vi "数据存储接口.vi"(4 "快捷测试？":bool, 5 "质控参数设置":T1, 6 "标样校准？":bool, 7 "数据标记表":string, 8 "空白校准？":bool, 10 "数据存储模式":T2(ring), 11 "测量数据区":T4) -> (2 "x != y?":bool, 3 "data输出":T3)   [LabVIEW 2016, in "斯坦道总磷总氮.lvlib"]
panel:
  # "跨度值"
  # "零点核查标准液浓度"
  # "跨度核查标准液浓度"
  # "标样核查标准液浓度"
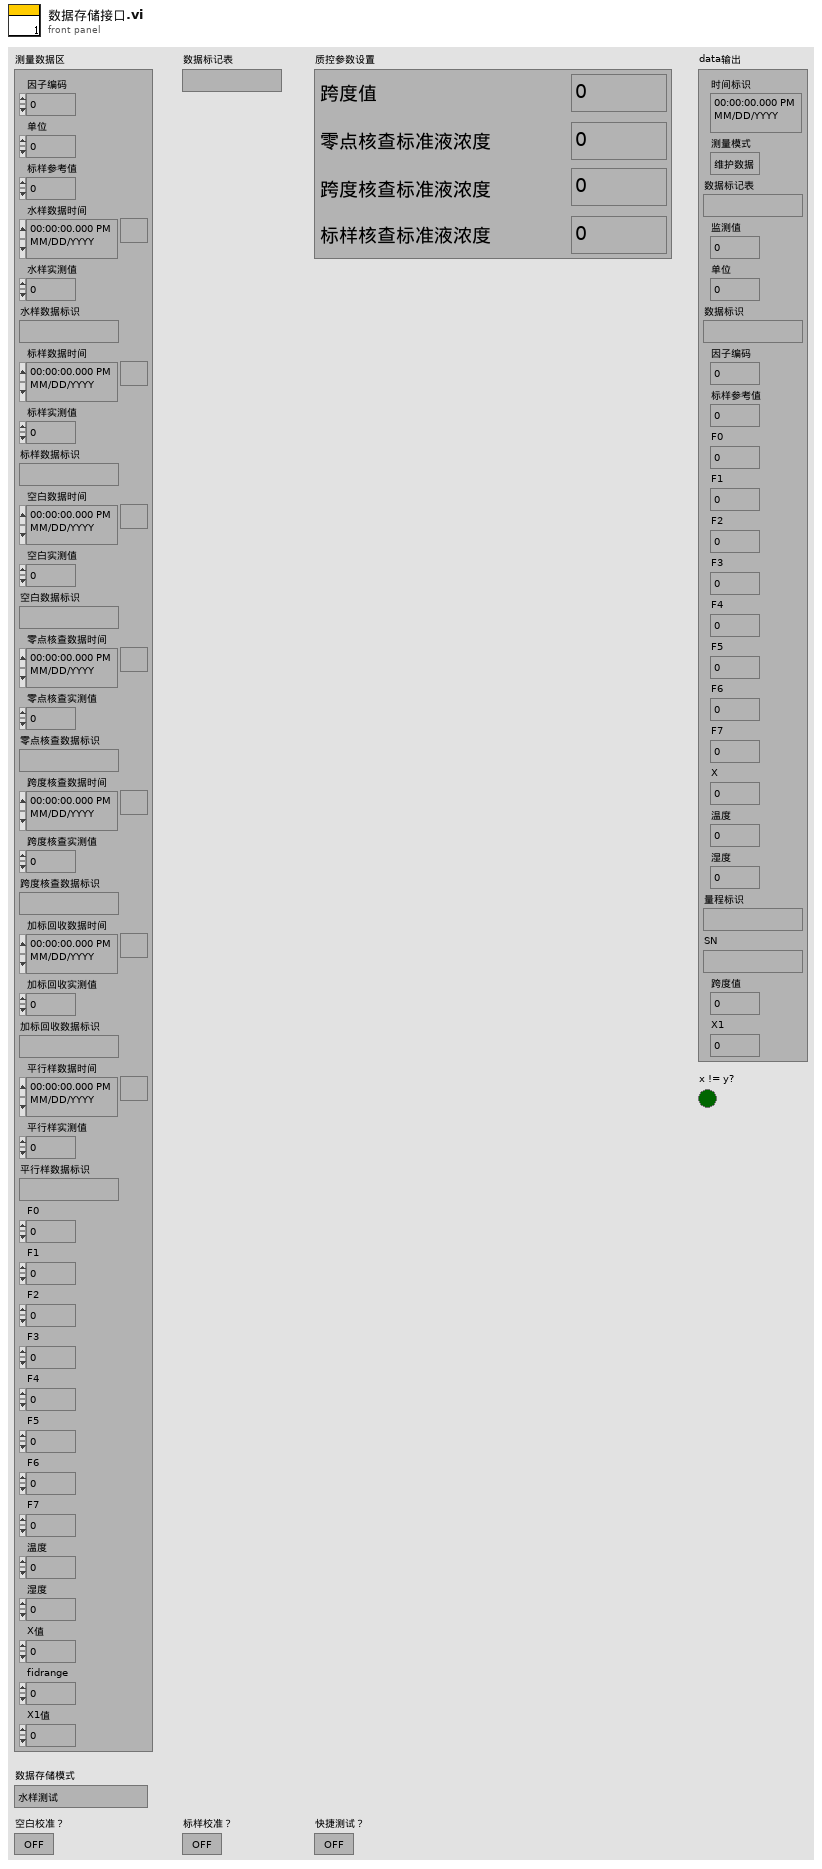
[diagram p1: front panel]
types:
  T1 = cluster{"跨度值":dbl, "零点标准液浓度":dbl, "跨度标准液浓度":dbl, "标准液标准浓度":dbl}
  T2 = enum16{"水样测试", "标样核查", "跨度核查", "零点核查", "加标回收", "空白测试", "平行样"}
  T3 = cluster{"时间标识":timestamp, "测量模式":enum16{"维护数据", "水样测试", "标样核查", "零点核查", "跨度核查", "空白测试", "平行样测试", "加标回收", "空白校准", "标样校准", "初始化（清洗）", "快捷测试"}, "数据标记表":string, "监测值":sgl, "单位":u16, "数据标识":string, "因子编码":u32, "标样参考值":sgl, "F0":sgl, "F1":sgl, "F2":sgl, "F3":sgl, "F4":sgl, "F5":sgl, "F6":sgl, "F7":sgl, "X":sgl, "温度":sgl, "湿度":sgl, "量程标识":string, "SN":string, "跨度值":sgl, "X1":sgl}
  T4 = cluster{"因子编码":u32, "单位":u16, "标样参考值":sgl, "水样数据时间":timestamp, "水样实测值":sgl, "水样数据标识":string, "标样数据时间":timestamp, "标样实测值":sgl, "标样数据标识":string, "空白数据时间":timestamp, "空白实测值":sgl, "空白数据标识":string, "零点核查数据时间":timestamp, "零点核查实测值":sgl, "零点核查数据标识":string, "跨度核查数据时间":timestamp, "跨度核查实测值":sgl, "跨度核查数据标识":string, "加标回收数据时间":timestamp, "加标回收实测值":sgl, "加标回收数据标识":string, "平行样数据时间":timestamp, "平行样实测值":sgl, "平行样数据标识":string, "F0":sgl, "F1":sgl, "F2":sgl, "F3":sgl, "F4":sgl, "F5":sgl, "F6":sgl, "F7":sgl, "温度":sgl, "湿度":sgl, "X值":sgl, "fidrange":u16, "X1值":sgl}
  T5 = enum16{"维护数据", "水样测试", "标样核查", "零点核查", "跨度核查", "空白测试", "平行样测试", "加标回收", "空白校准", "标样校准", "初始化（清洗）", "快捷测试"}
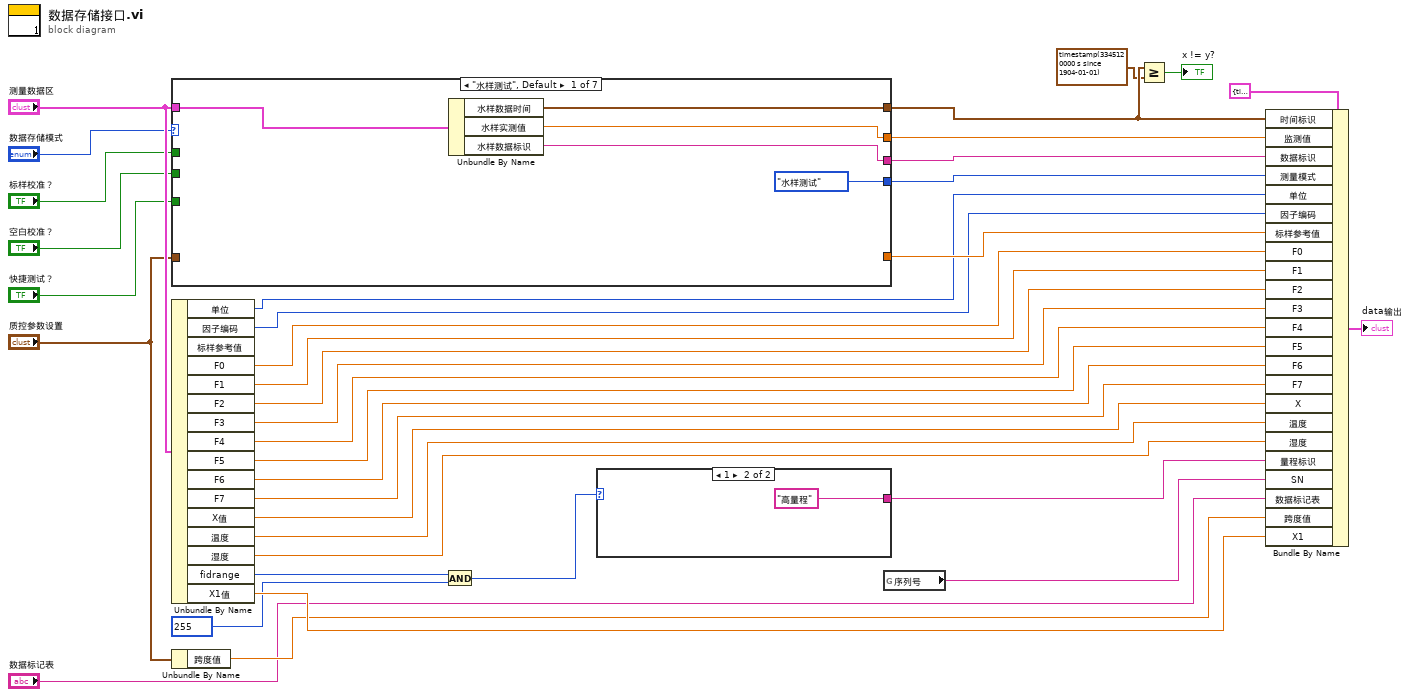
[diagram p0: block diagram]
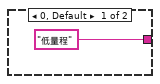
[diagram p2: hidden frame]
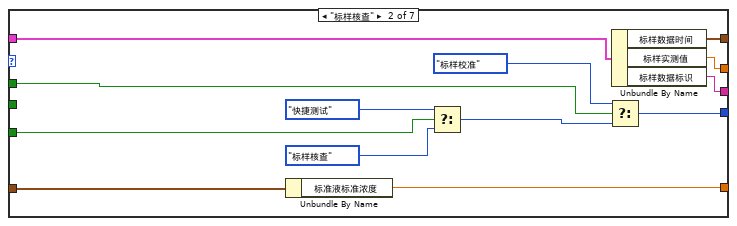
[diagram p3: hidden frame]
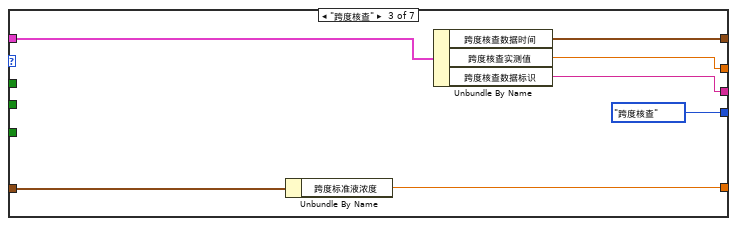
[diagram p4: hidden frame]
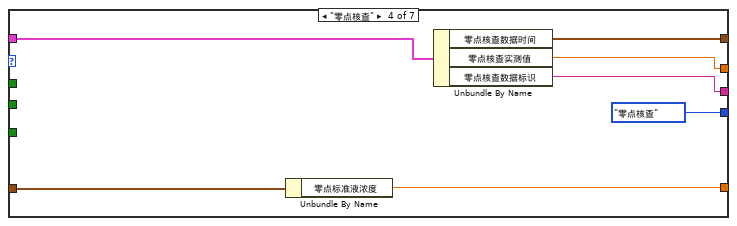
[diagram p5: hidden frame]
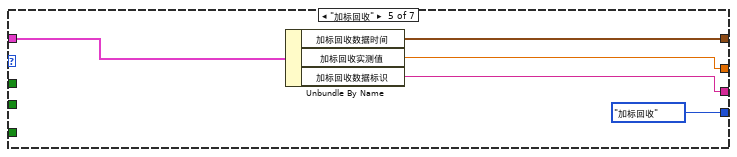
[diagram p6: hidden frame]
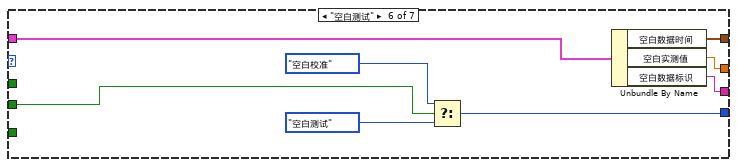
[diagram p7: hidden frame]
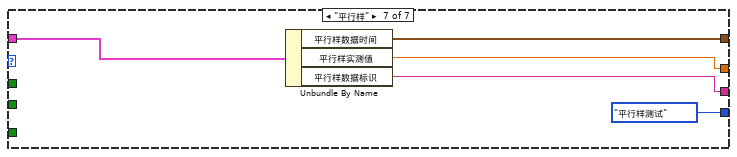
[diagram p8: hidden frame]
diagram:
  n1 = case shown="\"水样测试\", Default" "数据存储模式" {
    tunnel: "测量数据区" -> [w41 w54 w61 w68 w73 w81 w86]
    tunnel: [w40 w53 w60 w67 w72 w80 w85] -> w3
    tunnel: [w39 w52 w59 w66 w71 w79 w84] -> w23
    tunnel: [w38 w51 w58 w65 w70 w78 w83] -> w22
    tunnel: [T5."水样测试" ("测量模式") w44 T5."跨度核查" ("测量模式") T5."零点核查" ("测量模式") T5."加标回收" ("测量模式") w75 T5."平行样测试" ("测量模式")] -> w33
    tunnel: "质控参数设置" -> [_ w50 w57 w64 _ _ _]
    tunnel: [_ w49 w56 w63 _ _ _] -> w25
    tunnel: "空白校准？" -> [_ _ _ _ _ w74 _]
    tunnel: "标样校准？" -> [_ w43 _ _ _ _ _]
    tunnel: "快捷测试？" -> [_ w42 _ _ _ _ _]
    frame "水样测试", Default {
      n2 = Unbundle By Name(w41) -> ("水样数据时间"=w40:timestamp, "水样实测值"=w39:sgl, "水样数据标识"=w38:string)
    }
    frame "标样核查" {
      n3 = Unbundle By Name(w50) -> ("标准液标准浓度"=w49:dbl)
      n4 = Select(t=T5."快捷测试" ("测量模式"), s=w42, f=T5."标样核查" ("测量模式")) -> (s? t:f=w45:T5)
      n5 = Select(t=T5."标样校准" ("测量模式"), s=w43, f=w45) -> (s? t:f=w44:T5)
      n6 = Unbundle By Name(w54) -> ("标样数据时间"=w53:timestamp, "标样实测值"=w52:sgl, "标样数据标识"=w51:string)
    }
    frame "跨度核查" {
      n7 = Unbundle By Name(w57) -> ("跨度标准液浓度"=w56:dbl)
      n8 = Unbundle By Name(w61) -> ("跨度核查数据时间"=w60:timestamp, "跨度核查实测值"=w59:sgl, "跨度核查数据标识"=w58:string)
    }
    frame "零点核查" {
      n9 = Unbundle By Name(w64) -> ("零点标准液浓度"=w63:dbl)
      n10 = Unbundle By Name(w68) -> ("零点核查数据时间"=w67:timestamp, "零点核查实测值"=w66:sgl, "零点核查数据标识"=w65:string)
    }
    frame "加标回收" {
      n11 = Unbundle By Name(w73) -> ("加标回收数据时间"=w72:timestamp, "加标回收实测值"=w71:sgl, "加标回收数据标识"=w70:string)
    }
    frame "空白测试" {
      n12 = Select(t=T5."空白校准" ("测量模式"), s=w74, f=T5."空白测试" ("测量模式")) -> (s? t:f=w75:T5)
      n13 = Unbundle By Name(w81) -> ("空白数据时间"=w80:timestamp, "空白实测值"=w79:sgl, "空白数据标识"=w78:string)
    }
    frame "平行样" {
      n14 = Unbundle By Name(w86) -> ("平行样数据时间"=w85:timestamp, "平行样实测值"=w84:sgl, "平行样数据标识"=w83:string)
    }
  }
  n15 = Unbundle By Name("测量数据区") -> ("单位"=w9:u16, "因子编码"=w10:u32, "F0"=w11:sgl, "F1"=w12:sgl, "F2"=w13:sgl, "F3"=w14:sgl, "F4"=w15:sgl, "F5"=w16:sgl, "F6"=w17:sgl, "F7"=w18:sgl, "X值"=w19:sgl, "温度"=w20:sgl, "湿度"=w21:sgl, "fidrange"=w26:u16, "X1值"=w36:sgl)  [unwired: 1 out]
  n16 = Unbundle By Name("质控参数设置") -> ("跨度值"=w34:dbl)
  n17 = And(x=w26, y=u16 255) -> (x .and. y?=w28:u16)
  n18 = case shown="1" w28 {
    tunnel: ["低量程" ("格式字符串") "高量程" ("格式字符串")] -> w29
    frame 0, Default {
    }
    frame 1 {
    }
  }
  n19 = global read "VAR总磷总氮全局变量.vi" "序列号"() -> (w31:string)
  n20 = Greater Or Equal?(x=w3, y=timestamp(3345120000 s since 1904-01-01) ("x")) -> (x >= y?=→"x != y?":bool)
  n21 = Bundle By Name(cluster=T3 {"时间标识"=timestamp(0 s since 1904-01-01), "测量模式"=enum."维护数据", "数据标记表"="", "监测值"=0.0, "单位"=0, "数据标识"="", "因子编码"=0, "标样参考值"=0.0, "F0"=0.0, "F1"=0.0, "F2"=0.0, "F3"=0.0, "F4"=0.0, "F5"=0.0, "F6"=0.0, "F7"=0.0, "X"=0.0, "温度"=0.0, "湿度"=0.0, "量程标识"="", "SN"="", "跨度值"=0.0, "X1"=0.0} ("data输入"), "时间标识"=w3, "监测值"=w23, "数据标识"=w22, "测量模式"=w33, "单位"=w9, "因子编码"=w10, "标样参考值"=w25, "F0"=w11, "F1"=w12, "F2"=w13, "F3"=w14, "F4"=w15, "F5"=w16, "F6"=w17, "F7"=w18, "X"=w19, "温度"=w20, "湿度"=w21, "量程标识"=w29, "SN"=w31, "数据标记表"="数据标记表", "跨度值"=w34, "X1"=w36) -> (→"data输出":T3)
